vi "Camera Selector.vi"(8 "error in (no error)":errorcluster) -> (0 "error out":errorcluster, 3 "Image Acquisition out":refnum<class "Camera.lvclass">)   [LabVIEW 2019]
uses:
  Camera.lvclass
panel:
  in  "Choose Camera":string(combo)
  in  "OK Button":bool
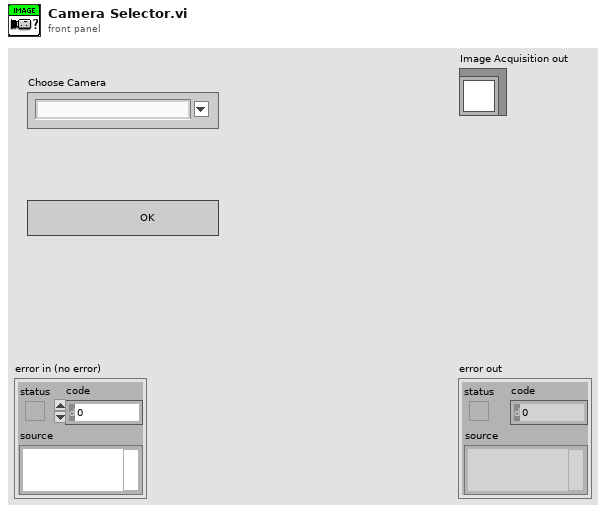
[diagram p1: front panel]
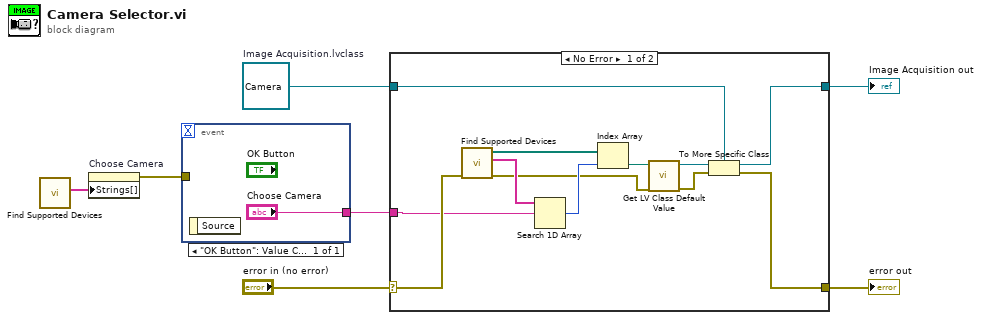
[diagram p0: block diagram]
diagram:
  w4 = refnum<class "Camera.lvclass"> refnum  # Image Acquisition.lvclass
  n1 = call "Find Supported Devices.vi"() -> ("Supported Cameras"=w3:string[])  [unwired: 9 in, 2 out]
  n2 = property on="Choose Camera" class="CmbBox"("Strings[]"=w3) -> (error out=w1:errorcluster)  [unwired: 2 in, 1 out]
  n3 = event shown="[0] \"OK Button\": Value Change" {
    selector: _ -> [_]
    dyn-events: _ -> [_]
    timeout: _ -> [_]
    tunnel: ["Choose Camera"] -> w2
    tunnel: w1 -> [_]
    event "OK Button": Value Change {
      n4 = event-data() -> ()  [unwired: 1 in, 1 out]
    }
  }
  n5 = case shown="No Error" "error in (no error)" {
    selector: "error in (no error)" -> [w12 w22]
    tunnel: [w18 w22] -> w6
    tunnel: [w17 w21] -> w5
    tunnel: w4 -> [w10 w21]
    tunnel: w2 -> [w9 _]
    frame No Error {
      n6 = call "Find Supported Devices.vi"("error in (no error)"=w12) -> ("error out"=w11:errorcluster, "Supported Cameras"=w16:string[], "Camera Driver Paths"=w15:path[])  [unwired: 8 in]
      n7 = Search 1D Array(1D array=w16, element=w9) -> (index of element=w14:i32)  [unwired: 1 in]
      n8 = Index Array(array=w15, index=w14) -> (element=w13:path)
      n9 = call <vilib>:"Get LV Class Default Value.vi"("error in (no error)"=w11, "class path"=w13) -> ("error out"=w19:errorcluster, "object"=w20:refnum<class>)  [unwired: 8 in]
      n10 = To More Specific Class(target class=w10, reference=w20, error in=w19) -> (specific class reference=w17:refnum<class "Camera.lvclass">, error out=w18:errorcluster)
    }
    frame Error {
    }
  }
  "error out" <- w6
  "Image Acquisition out" <- w5
